vi "4-1.vi"() -> ()   [LabVIEW 2019, in "4.lvlib"]
uses:
  4.lvlib
panel:
  out "Bingo":i32
  out "Array":i32[](array[numeric])
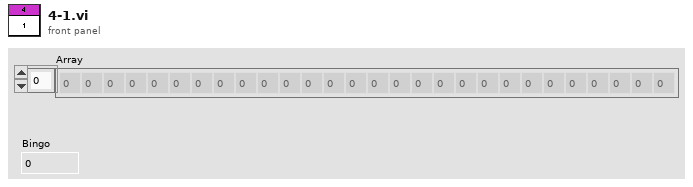
[diagram p1: front panel]
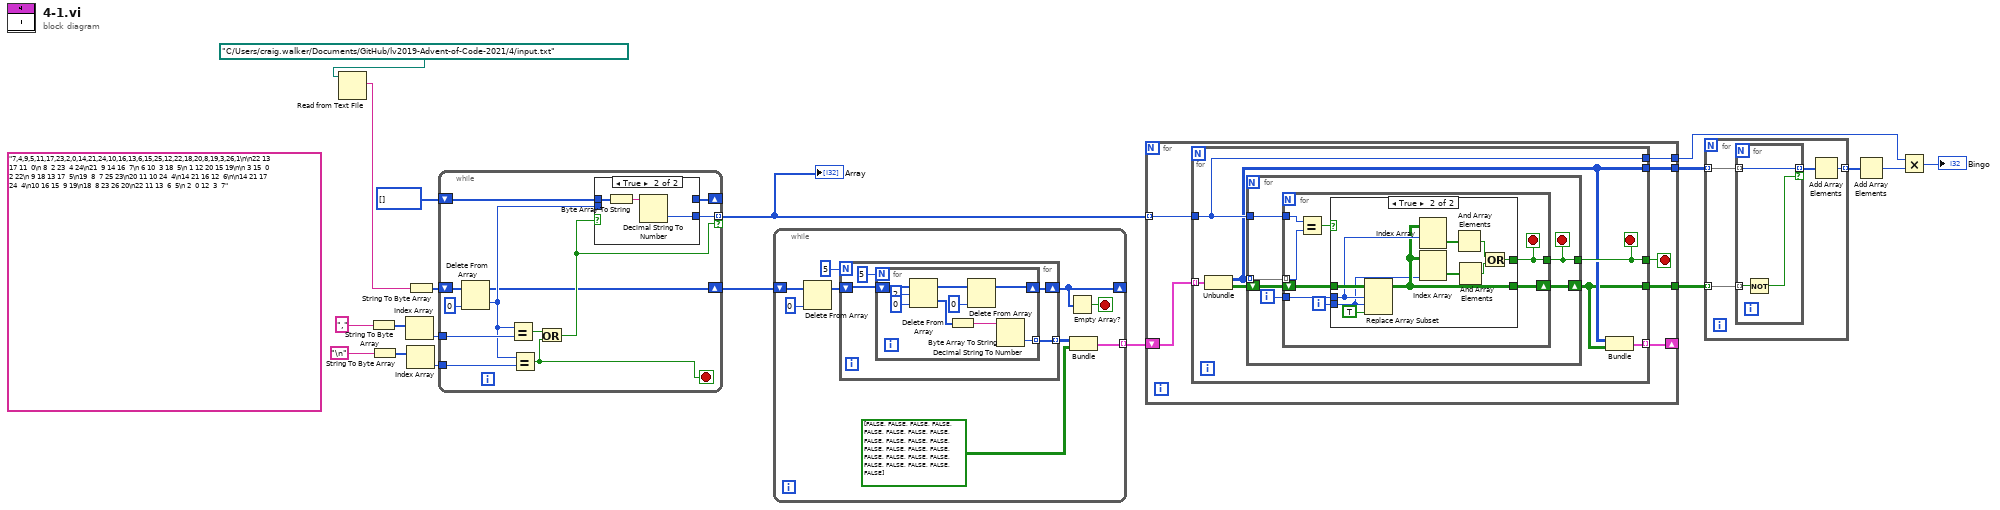
[diagram p0: block diagram]
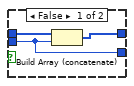
[diagram p3: hidden frame]
diagram:
  (unwired) "7,4,9,5,11,17,23,2,0,14,21,24,10,16,13,6,15,25,12,22,18,20,8,19,3,26,1\n\n22 13 17 11  0\n 8  2 23  4 24\n21  9 14 16  7\n 6 10  3 18  5\n 1 12 20 15 19\n\n 3 15  0  2 22\n 9 18 13 17  5\n19  8  7 25 23\n20 11 10 24  4\n14 21 16 12  6\n\n14 21 17 24  4\n10 16 15  9 19\n18  8 23 26 20\n22 11 13  6  5\n 2  0 12  3  7"
  n1 = Read from Text File(file (use dialog)=path "C:/Users/craig.walker/Documents/GitHub/lv2019-Advent-of-Code-2021/4/input.txt" ("file path (dialog if empty)")) -> (text=w1:string)  [unwired: 3 in, 3 out]
  n2 = String To Byte Array(string="," ("delimiter (Tab)")) -> (unsigned byte array=w18:u8[])
  n3 = String To Byte Array(string="\n") -> (unsigned byte array=w15:u8[])
  n4 = Index Array(array=w18) -> (element=w17:u8)  [unwired: 1 in]
  n5 = Index Array(array=w15) -> (element=w13:u8)  [unwired: 1 in]
  n6 = String To Byte Array(string=w1) -> (unsigned byte array=w12:u8[])
  n7 = while {
    tunnel: w17 -> [w29]
    shift-right: [w30] -> _
    shift-left: u8[] [] ("disabled index (col)") -> [w31]
    tunnel: [w28] -> w8 mode=indexing if=w24
    tunnel: w13 -> [w27]
    shift-right: [w21] -> w11
    shift-left: w12 -> [w26]
    stop <- w23 stop-if-true
    n8 = Delete From Array(array=w26, index=0) -> (deleted portion=w22:u8, array with subset deleted=w21:u8[])  [unwired: 1 in]
    n9 = Equal?(x=w22, y=w29) -> (x = y?=w25:bool)
    n10 = Equal?(x=w22, y=w27) -> (x = y?=w23:bool)
    n11 = Or(x=w25, y=w23) -> (x .or. y?=w24:bool)
    n12 = case shown="True" w24 {
      tunnel: w31 -> [w34 w37]
      tunnel: [w33 _] -> w30
      tunnel: w22 -> [w32 _]
      tunnel: [w32 w35] -> w28
      frame False {
        n13 = Build Array (concatenate)(w34, w32) -> (w33:u8[])
      }
      frame True {
        n14 = Byte Array To String(unsigned byte array=w37) -> (string=w36:string)
        n15 = Decimal String To Number(string=w36) -> (number=w35:i32)  [unwired: 2 in, 1 out]
      }
    }
  }
  "Array" <- w8
  n16 = while {
    shift-right: [w40] -> _
    shift-left: w11 -> [w46]
    tunnel: [w41] -> w9 mode=indexing
    stop <- w39 stop-if-true
    n17 = Delete From Array(array=w46, index=0) -> (array with subset deleted=w43:u8[])  [unwired: 1 in, 1 out]
    n18 = for {
      N: 5 -> [_]
      tunnel: [w48] -> w42 mode=indexing
      shift-right: [w47] -> w40
      shift-left: w43 -> [w50]
      n19 = for {
        N: 5 -> [_]
        tunnel: [w52] -> w48 mode=indexing
        shift-right: [w51] -> w47
        shift-left: w50 -> [w59]
        n20 = Delete From Array(array=w59, length=2, index=0) -> (deleted portion=w54:u8[], array with subset deleted=w56:u8[])
        n21 = Byte Array To String(unsigned byte array=w54) -> (string=w53:string)
        n22 = Delete From Array(array=w56, index=0) -> (array with subset deleted=w51:u8[])  [unwired: 1 in, 1 out]
        n23 = Decimal String To Number(string=w53) -> (number=w52:i32)  [unwired: 2 in, 1 out]
      }
    }
    n24 = Empty Array?(array=w40) -> (empty?=w39:bool)
    n25 = Bundle(w42, bool[][] [[FALSE, FALSE, FALSE, FALSE, FALSE], [FALSE, FALSE, FALSE, FALSE, FALSE], [FALSE, FALSE, FALSE, FALSE, FALSE], [FALSE, FALSE, FALSE, FALSE, FALSE], [FALSE, FALSE, FALSE, FALSE, FALSE]]) -> (w41:cluster{i32[][], bool[][]})  [unwired: 1 in]
  }
  n26 = for {
    tunnel: w8 -> [w65] mode=indexing
    tunnel: [w64] -> w3
    tunnel: [w63] -> w6
    tunnel: [w61] -> w7
    shift-right: [w60] -> _
    shift-left: w9 -> [w66]
    stop <- w62 stop-if-true
    n27 = for {
      tunnel: w66 -> [w73] mode=indexing
      tunnel: w65 -> [w71]
      tunnel: [w69] -> w63
      tunnel: [w71] -> w64
      tunnel: [w70] -> w62
      tunnel: [w68] -> w61
      tunnel: [w67] -> w60 mode=indexing
      stop <- w70 stop-if-true
      n28 = Unbundle(w73) -> (w69:i32[][], w72:bool[][])
      n29 = for {
        tunnel: w69 -> [w76] mode=indexing
        tunnel: w71 -> [w78]
        tunnel: [w75] -> w70
        shift-right: [w74] -> w68
        shift-left: w72 -> [w79]
        i -> [w77]
        stop <- w75 stop-if-true
        n30 = for {
          tunnel: w76 -> [w86] mode=indexing
          tunnel: w78 -> [w85]
          tunnel: w77 -> [w83]
          tunnel: [w81] -> w75
          shift-right: [w80] -> w74
          shift-left: w79 -> [w84]
          i -> [w82]
          stop <- w81 stop-if-true
          n31 = Equal?(x=w85, y=w86) -> (x = y?=w87:bool)
          n32 = case shown="True" w87 {
            tunnel: w84 -> [w88 w98]
            tunnel: w83 -> [_ w96]
            tunnel: w82 -> [_ w93]
            tunnel: [w88 w94] -> w80
            tunnel: [_ w89] -> w81
            frame False {
            }
            frame True {
              n33 = Replace Array Subset(array=w98, new element=TRUE ("new element/subarray"), index (row)=w96, index (col)=w93) -> (w94:bool[][])
              n34 = Index Array(array=w94, index (row)=w96) -> (element=w95:bool[])  [unwired: 1 in]
              n35 = Index Array(array=w94, index (col)=w93) -> (element=w92:bool[])  [unwired: 1 in]
              n36 = And Array Elements(Boolean array=w95) -> (logical AND=w90:bool)
              n37 = And Array Elements(Boolean array=w92) -> (logical AND=w91:bool)
              n38 = Or(x=w90, y=w91) -> (x .or. y?=w89:bool)
            }
          }
        }
      }
      n39 = Bundle(w69, w68) -> (w67:cluster{i32[][], bool[][]})  [unwired: 1 in]
    }
  }
  n40 = for {
    tunnel: w7 -> [w102] mode=indexing
    tunnel: w6 -> [w101] mode=indexing
    tunnel: [w99] -> w5 mode=indexing
    n41 = for {
      tunnel: w102 -> [w104] mode=indexing
      tunnel: w101 -> [w105] mode=indexing
      tunnel: [w105] -> w100 mode=indexing if=w103
      n42 = Not(x=w104) -> (.not. x?=w103:bool)
    }
    n43 = Add Array Elements(numeric array=w100) -> (sum=w99:i32)
  }
  n44 = Add Array Elements(numeric array=w5) -> (sum=w4:i32)
  n45 = Multiply(x=w3, y=w4) -> (x*y=→"Bingo":i32)
